vi "Write Data average.vi"(8 "error in (no error)":errorcluster, 11 "DATA in":refnum<class "DATA.lvclass">) -> (0 "error out":errorcluster, 3 "DATA out":refnum<class "DATA.lvclass">)   [LabVIEW 2019, in "DATA.lvclass"]
uses:
  DATA.lvclass
  DATA.lvclass/DATA.ctl
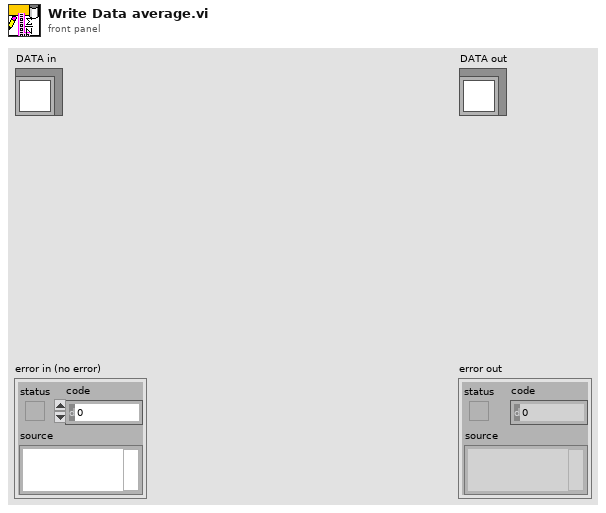
[diagram p1: front panel]
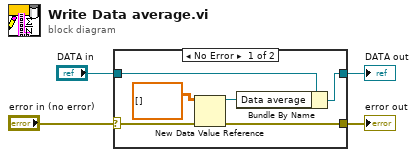
[diagram p0: block diagram]
diagram:
  n1 = case shown="No Error" "error in (no error)" {
    selector: "error in (no error)" -> [w8 w11]
    tunnel: [w7 w11] -> w3
    tunnel: [w10 w12] -> w1
    tunnel: "DATA in" -> [w5 w12]
    frame No Error {
      n2 = New Data Value Reference(data value=dbl[][] [] ("appended array"), error in=w8) -> (data value reference=w6:refnum<data-value>, error out=w7:errorcluster)
      n3 = Bundle By Name(cluster=w5, "Data average"=w6) -> (w10:refnum<class "DATA.lvclass">)
    }
    frame Error {
    }
  }
  "error out" <- w3
  "DATA out" <- w1
